vi "jsonToLibera.vi"(0 "json":string, 1 "Enable DD":bool, 3 "Enable SA":bool, 4 "Enable ADC CW":bool, 10 "Enable ADC SP":bool, 11 "Enable AVG":bool) -> (5 "STATUS":string, 6 "ADC_CW":T1(array[cluster]), 7 "AVG":cluster{"AVG":i32}[](array[cluster]), 8 "ST":u64, 9 "MT":u64, 12 "DD":T5(array[cluster]), 13 "SA":T3(array[cluster]), 14 "mode":i32, 15 "acquisitions":string, 16 "samples":i32, 17 "libera_error":i32, 19 "ADC_SP":T2(array[cluster]))   [LabVIEW 2014]
uses:
  common/crest/LabVIEW/LV14/chaosui-crest/chaosui-crest.lvlib
panel:
  out "value":T4
  out "nok":i32
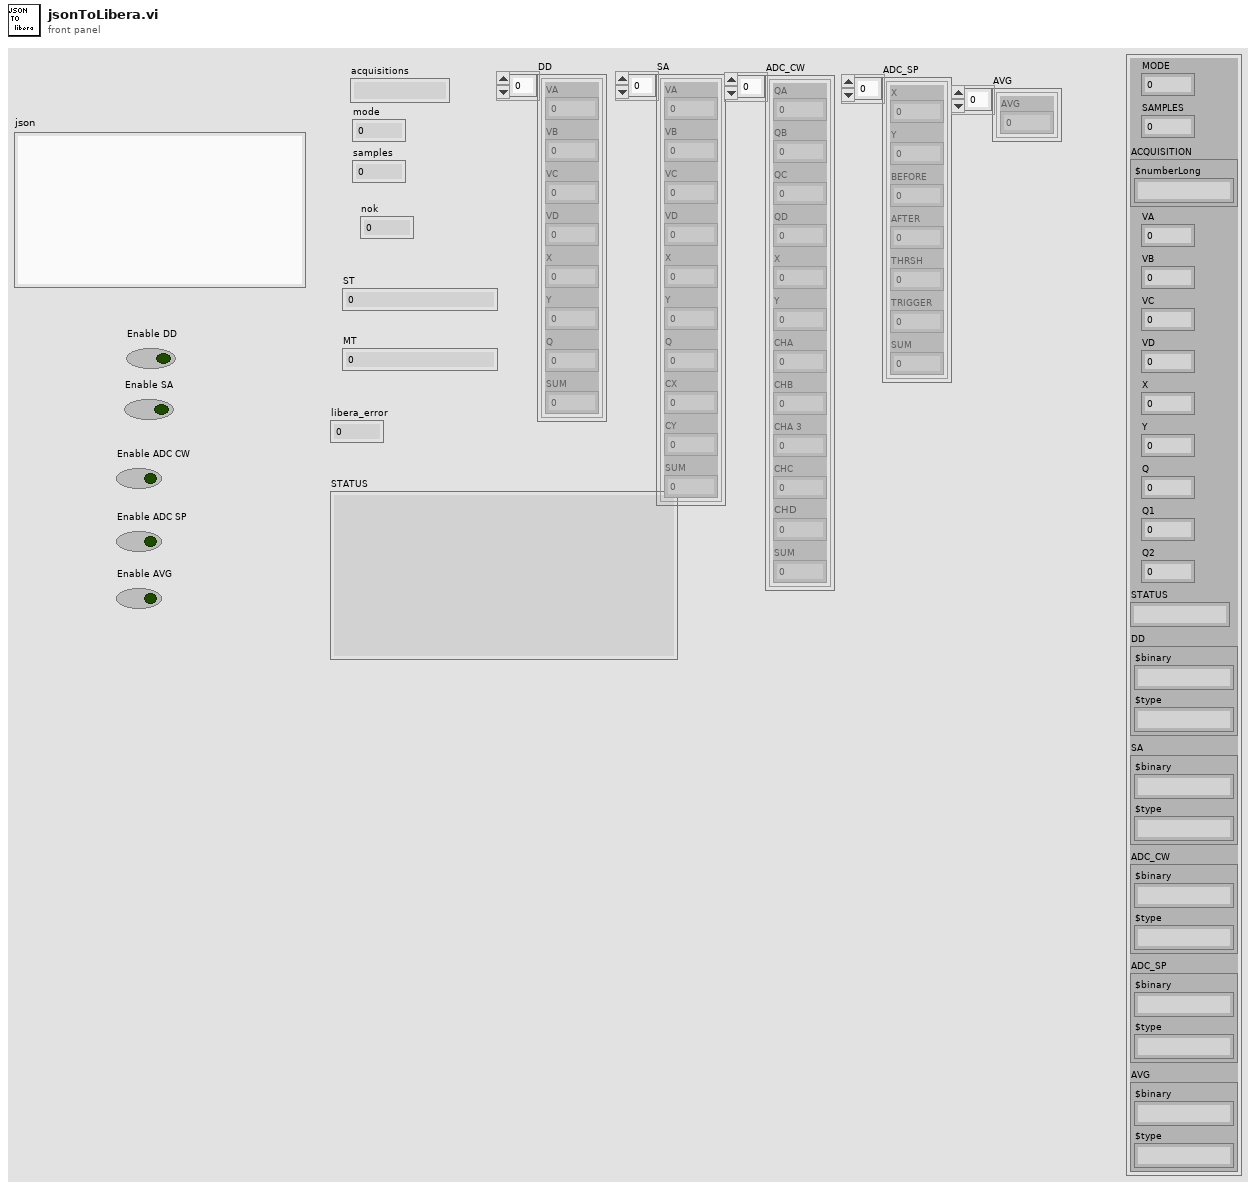
[diagram p1: front panel]
types:
  T1 = cluster{"QA":i32, "QB":i32, "QC":i32, "QD":i32, "X":i32, "Y":i32, "CHA":i32, "CHB":i32, "CHA 3":i32, "CHC":i32, "CHD":i32, "SUM":i32}[]
  T2 = cluster{"X":i32, "Y":i32, "BEFORE":i32, "AFTER":i32, "THRSH":i32, "TRIGGER":i32, "SUM":i32}[]
  T3 = cluster{"VA":i32, "VB":i32, "VC":i32, "VD":i32, "X":i32, "Y ":i32, "Q":i32, "CX":i32, "CY":i32, "SUM":i32}[]
  T4 = cluster{"MODE":i32, "SAMPLES":i32, "ACQUISITION":cluster{"$numberLong":string}, "VA":i32, "VB":i32, "VC":i32, "VD":i32, "X":i32, "Y ":i32, "Q":i32, "Q1":i32, "Q2":i32, "STATUS":string, "DD":cluster{"$binary":string, "$type":string}, "SA":cluster{"$binary":string, "$type":string}, "ADC_CW":cluster{"$binary":string, "$type":string}, "ADC_SP":cluster{"$binary":string, "$type":string}, "AVG":cluster{"$binary":string, "$type":string}}
  T5 = cluster{"VA":i32, "VB":i32, "VC":i32, "VD":i32, "X":i32, "Y ":i32, "Q":i32, "SUM":i32}[]
  T6 = cluster{"MODE":i32, "SAMPLES":i32, "VA":i32, "VB":i32, "VC":i32, "VD":i32, "X":i32, "Y":i32, "ACQUISITION":cluster{"$numberLong":string}, "Q":i32, "STATUS":string, "Q1":i32, "Q2":i32, "DD":cluster{"$binary":string, "$type":string}, "SA":cluster{"$binary":string, "$type":string}, "ADC_CW":cluster{"$binary":string, "$type":string}, "ADC_SP":cluster{"$binary":string, "$type":string}, "AVG":cluster{"$binary":string, "$type":string}, "error":i32, "MT":cluster{"$numberLong":string}, "ST":cluster{"$numberLong":string}}
  T7 = enum16{"big-endian, network order", "native, host order", "little-endian"}
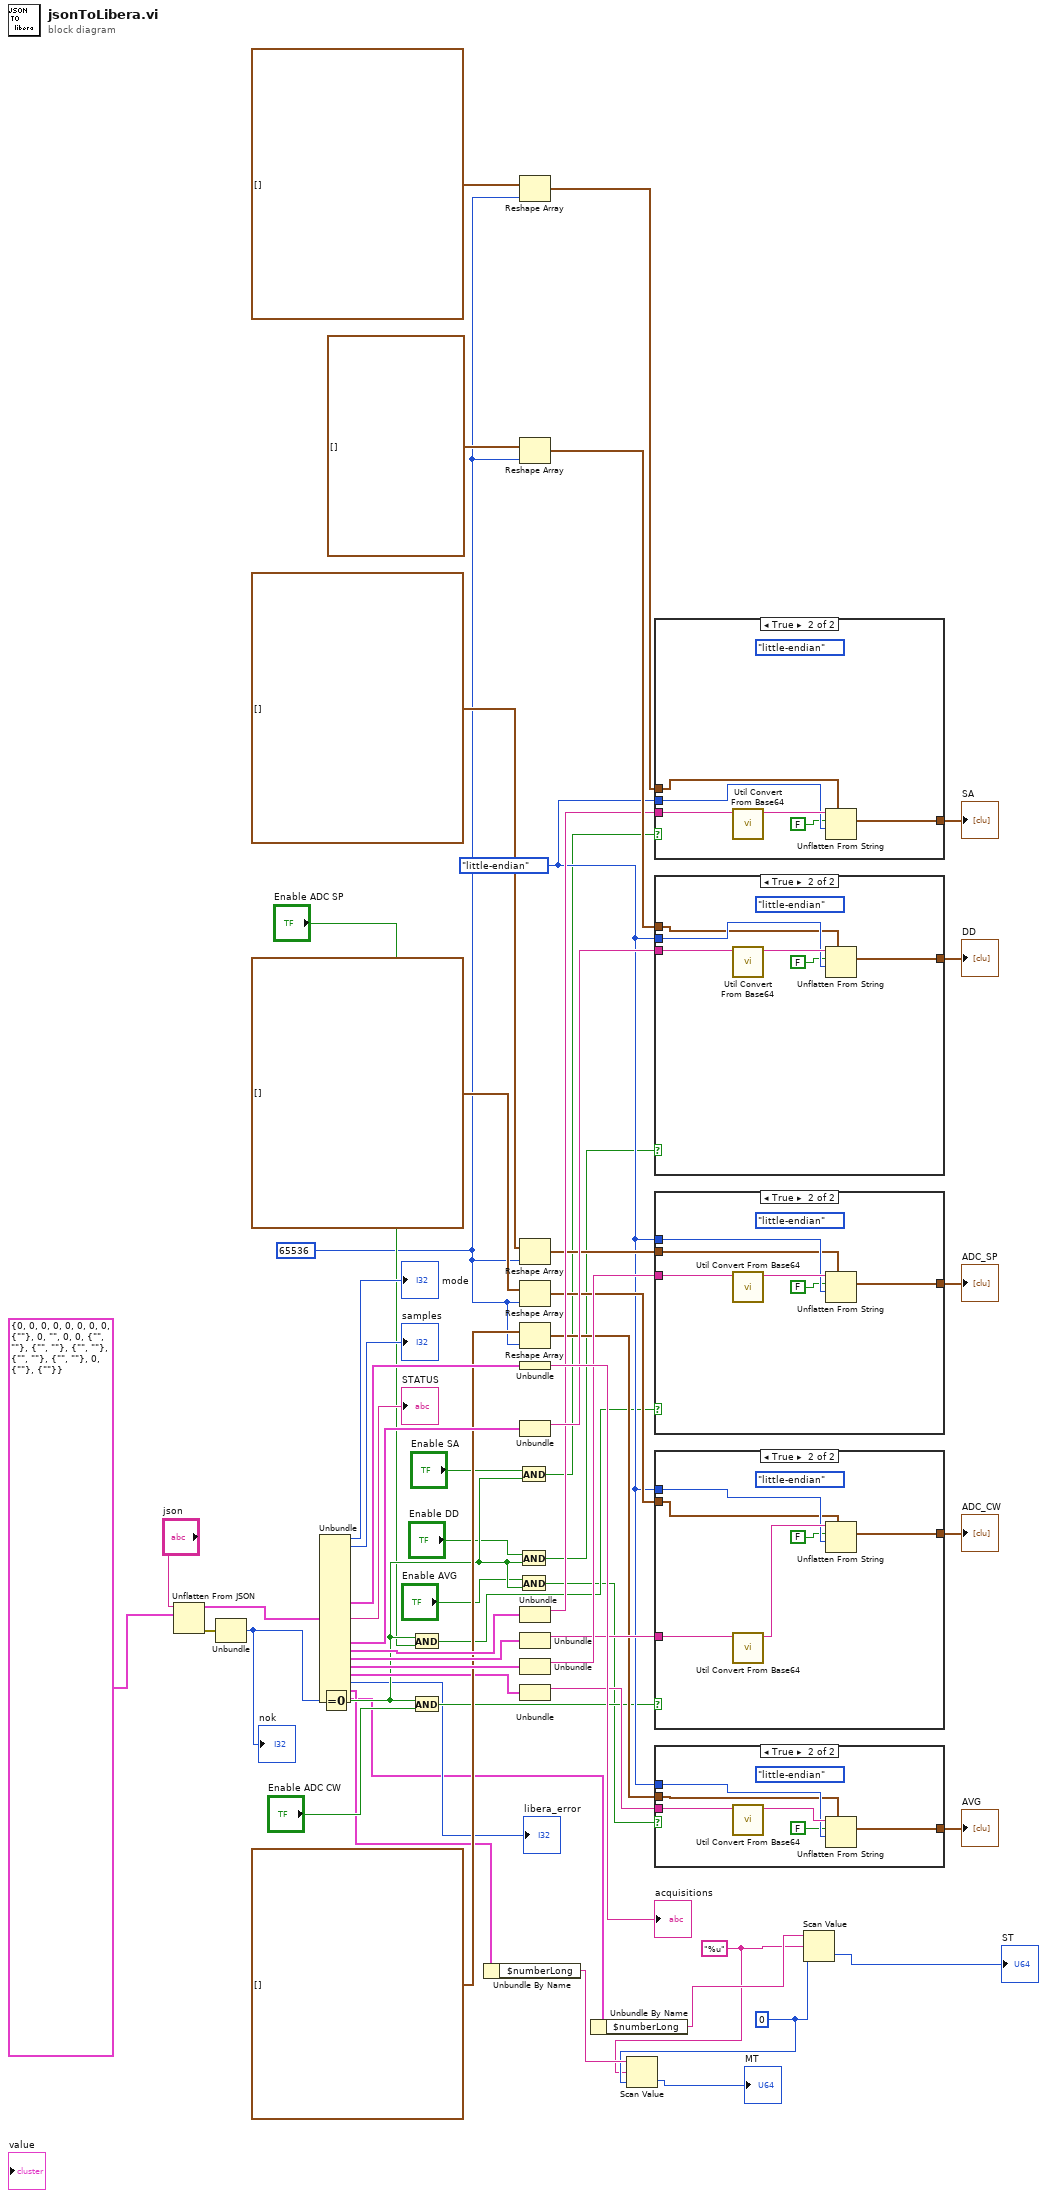
[diagram p0: block diagram]
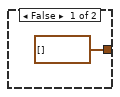
[diagram p2: hidden frame]
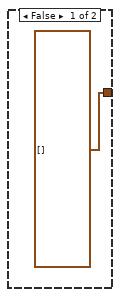
[diagram p3: hidden frame]
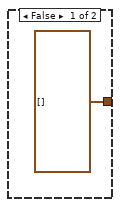
[diagram p4: hidden frame]
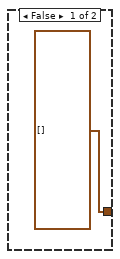
[diagram p5: hidden frame]
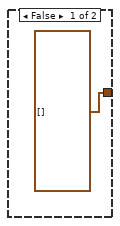
[diagram p6: hidden frame]
diagram:
  w1 = "%u" ("format string")
  w3 = u64 0
  w10 = 65536 ("dimension size")
  w26 = T7."little-endian" ("byte order (0:big-endian, network order)")
  n1 = Unflatten From JSON(JSON string="json", type and defaults=T6 {"MODE"=0, "SAMPLES"=0, "VA"=0, "VB"=0, "VC"=0, "VD"=0, "X"=0, "Y"=0, "ACQUISITION"={"$numberLong"=""}, "Q"=0, "STATUS"="", "Q1"=0, "Q2"=0, "DD"={"$binary"="", "$type"=""}, "SA"={"$binary"="", "$type"=""}, "ADC_CW"={"$binary"="", "$type"=""}, "ADC_SP"={"$binary"="", "$type"=""}, "AVG"={"$binary"="", "$type"=""}, "error"=0, "MT"={"$numberLong"=""}, "ST"={"$numberLong"=""}} ("jsonCluster")) -> (value=w55:T6, error out=w56:errorcluster)  [unwired: 5 in]
  n2 = Unbundle(w56) -> ("code"=w52:i32)  [unwired: 2 out]
  "nok" <- w52
  n3 = Unbundle(w55) -> ("MODE"=→"mode":i32, "SAMPLES"=→"samples":i32, "ACQUISITION"=w50:cluster{"$numberLong":string}, "STATUS"=→"STATUS":string, "DD"=w48:cluster{"$binary":string, "$type":string}, "SA"=w43:cluster{"$binary":string, "$type":string}, "ADC_CW"=w30:cluster{"$binary":string, "$type":string}, "ADC_SP"=w36:cluster{"$binary":string, "$type":string}, "AVG"=w25:cluster{"$binary":string, "$type":string}, "error"=→"libera_error":i32, "MT"=w8:cluster{"$numberLong":string}, "ST"=w7:cluster{"$numberLong":string})  [unwired: 9 out]
  n4 = Equal To 0?(x=w52) -> (x = 0?=w21:bool)
  n5 = And(x=w21, y="Enable ADC SP") -> (x .and. y?=w16:bool)
  n6 = And(x=w21, y="Enable ADC CW") -> (x .and. y?=w14:bool)
  n7 = Unbundle By Name(w8) -> ("$numberLong"=w4:string)
  n8 = And(x="Enable SA", y=w21) -> (x .and. y?=w20:bool)
  n9 = And(x="Enable DD", y=w21) -> (x .and. y?=w18:bool)
  n10 = And(x="Enable AVG", y=w21) -> (x .and. y?=w12:bool)
  n11 = Reshape Array(T3 [], w10) -> (w40:T3)
  n12 = Reshape Array(T5 [], w10) -> (w45:T5)
  n13 = Reshape Array(T2 [], w10) -> (w38:T2)
  n14 = Reshape Array(T1 [], w10) -> (w33:T1)
  n15 = Reshape Array(cluster{"AVG":i32}[] [], w10) -> (w28:cluster{"AVG":i32}[])
  n16 = Unbundle(w50) -> ("$numberLong"=→"acquisitions":string)
  n17 = Unbundle(w48) -> ("$binary"=w47:string)  [unwired: 1 out]
  n18 = Unbundle(w43) -> ("$binary"=w42:string)  [unwired: 1 out]
  n19 = Unbundle(w30) -> ("$binary"=w32:string)  [unwired: 1 out]
  n20 = Unbundle(w36) -> ("$binary"=w35:string)  [unwired: 1 out]
  n21 = Unbundle(w25) -> ("$binary"=w24:string)  [unwired: 1 out]
  n22 = Unbundle By Name(w7) -> ("$numberLong"=w6:string)
  n23 = Scan Value(string=w4, format string=w1, default (0 dbl)=w3) -> (value=→"MT":u64)  [unwired: 1 out]
  n24 = case shown="True" w20 {
    tunnel: w26 -> [_ w63]
    tunnel: w40 -> [_ w62]
    tunnel: [T3 [] w61] -> w39
    tunnel: w42 -> [_ w59]
    frame False {
    }
    frame True {
      (unwired) T7."little-endian" ("byte order (0:big-endian, network order)")
      n25 = call "Util Convert From Base64.vi"("Base64 String"=w59) -> ("String"=w64:string)  [unwired: 9 in, 1 out]
      n26 = Unflatten From String(type=w62, binary string=w64, data includes array or string size? (T)=FALSE, byte order (0:big-endian, network order)=w63) -> (value=w61:T3)  [unwired: 1 in, 2 out]
    }
  }
  "SA" <- w39
  n27 = case shown="True" w18 {
    tunnel: w26 -> [_ w70]
    tunnel: w45 -> [_ w69]
    tunnel: [T5 [] w68] -> w53
    tunnel: w47 -> [_ w67]
    frame False {
    }
    frame True {
      (unwired) T7."little-endian" ("byte order (0:big-endian, network order)")
      n28 = call "Util Convert From Base64.vi"("Base64 String"=w67) -> ("String"=w71:string)  [unwired: 9 in, 1 out]
      n29 = Unflatten From String(type=w69, binary string=w71, data includes array or string size? (T)=FALSE, byte order (0:big-endian, network order)=w70) -> (value=w68:T5)  [unwired: 1 in, 2 out]
    }
  }
  "DD" <- w53
  n30 = case shown="True" w16 {
    tunnel: w26 -> [_ w77]
    tunnel: w38 -> [_ w76]
    tunnel: w35 -> [_ w74]
    tunnel: [T2 [] w73] -> w34
    frame False {
    }
    frame True {
      (unwired) T7."little-endian" ("byte order (0:big-endian, network order)")
      n31 = call "Util Convert From Base64.vi"("Base64 String"=w74) -> ("String"=w78:string)  [unwired: 9 in, 1 out]
      n32 = Unflatten From String(type=w76, binary string=w78, data includes array or string size? (T)=FALSE, byte order (0:big-endian, network order)=w77) -> (value=w73:T2)  [unwired: 1 in, 2 out]
    }
  }
  "ADC_SP" <- w34
  n33 = case shown="True" w14 {
    tunnel: w26 -> [_ w84]
    tunnel: w33 -> [_ w83]
    tunnel: w32 -> [_ w81]
    tunnel: [T1 [] w80] -> w29
    frame False {
    }
    frame True {
      (unwired) T7."little-endian" ("byte order (0:big-endian, network order)")
      n34 = call "Util Convert From Base64.vi"("Base64 String"=w81) -> ("String"=w85:string)  [unwired: 9 in, 1 out]
      n35 = Unflatten From String(type=w83, binary string=w85, data includes array or string size? (T)=FALSE, byte order (0:big-endian, network order)=w84) -> (value=w80:T1)  [unwired: 1 in, 2 out]
    }
  }
  "ADC_CW" <- w29
  n36 = case shown="True" w12 {
    tunnel: w26 -> [_ w91]
    tunnel: w28 -> [_ w90]
    tunnel: w24 -> [_ w88]
    tunnel: [cluster{"AVG":i32}[] [] w87] -> w23
    frame False {
    }
    frame True {
      (unwired) T7."little-endian" ("byte order (0:big-endian, network order)")
      n37 = call "Util Convert From Base64.vi"("Base64 String"=w88) -> ("String"=w92:string)  [unwired: 9 in, 1 out]
      n38 = Unflatten From String(type=w90, binary string=w92, data includes array or string size? (T)=FALSE, byte order (0:big-endian, network order)=w91) -> (value=w87:cluster{"AVG":i32}[])  [unwired: 1 in, 2 out]
    }
  }
  "AVG" <- w23
  n39 = Scan Value(string=w6, format string=w1, default (0 dbl)=w3) -> (value=→"ST":u64)  [unwired: 1 out]
